vi "dll_driver.vi"(4 "position_llh":string="36.318462,138.996902,100", 6 "buffer size":i32=200000, 7 "dll state":T1(ring), 8 "error in":errorcluster, 9 "params":string, 10 "Rinex file":path=path "C:/Users/duyga/OneDrive/デスクトップ/WORKS/Nissan GPS/build dll/brdc0010.22n", 11 "dll Path":path=path "C:/Users/duyga/OneDrive/デスクトップ/WORKS/Nissan GPS/build dll/GPS_SIM_GENERATE_IQ.dll") -> (0 "error out":errorcluster, 3 "output":i16[](array[numeric]))   [LabVIEW 2020]
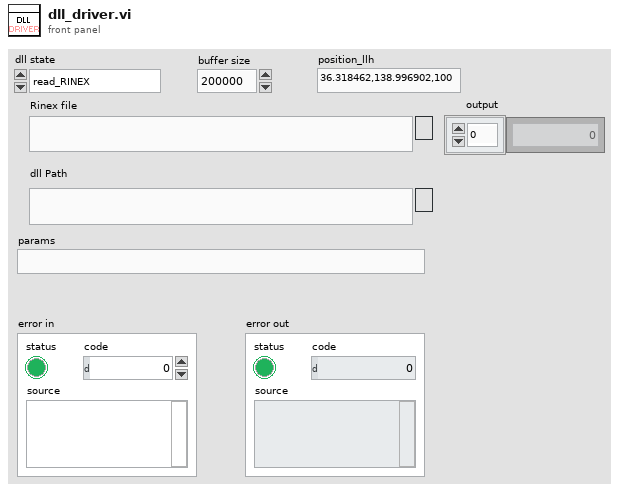
[diagram p1: front panel]
types:
  T1 = enum16{"read_RINEX", "settings", "generate_100ms", "update_position"}
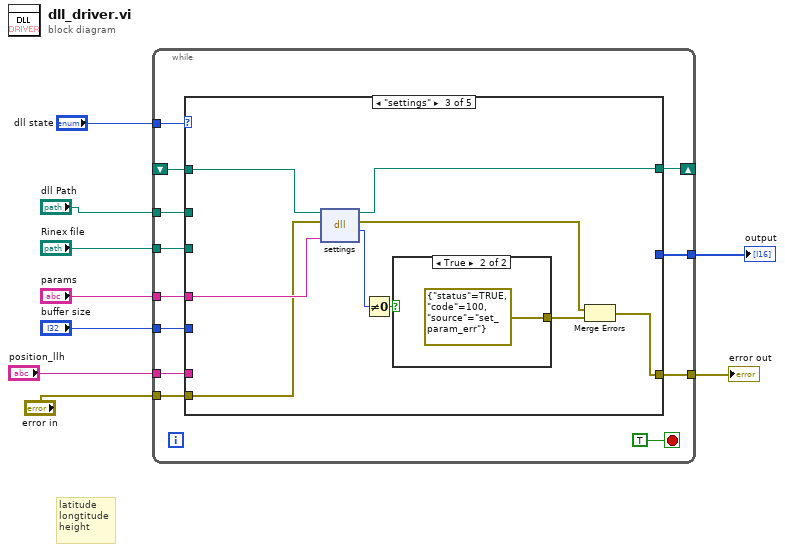
[diagram p0: block diagram]
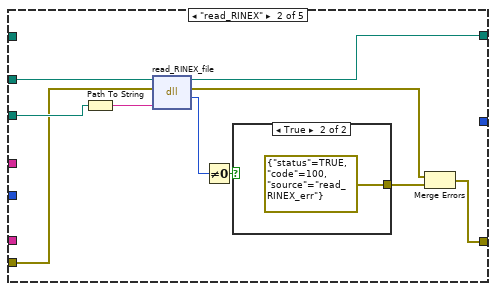
[diagram p3: hidden frame]
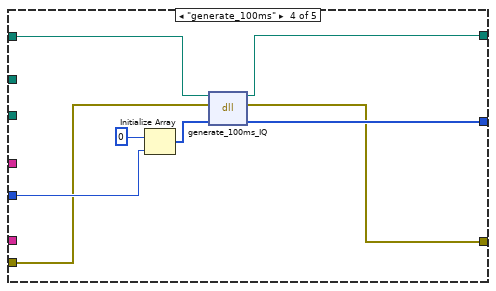
[diagram p6: hidden frame]
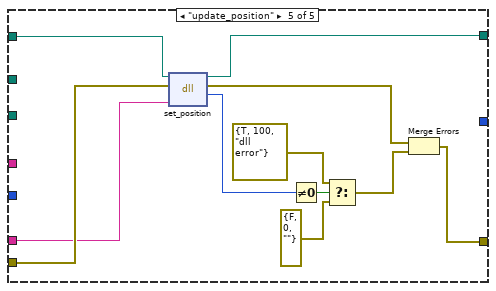
[diagram p7: hidden frame]
diagram:
  # "latitude\nlongtitude\nheight"
  n1 = while {
    tunnel: "dll state" -> [w20]
    tunnel: "dll Path" -> [w19]
    tunnel: "Rinex file" -> [w18]
    shift-right: [w17] -> _
    shift-left: _ -> [w14]
    tunnel: "error in" -> [w16]
    tunnel: [w15] -> w5
    tunnel: "params" -> [w13]
    tunnel: [w12] -> w3
    tunnel: "buffer size" -> [w11]
    tunnel: "position_llh" -> [w10]
    stop <- TRUE stop-if-true
    n2 = case shown="\"settings\"" w20 {
      tunnel: w19 -> [_ w32 _ _ _]
      tunnel: w18 -> [_ w31 _ _ _]
      tunnel: [w23 w30 w42 w47 w62] -> w17
      tunnel: w16 -> [w22 w29 w40 w45 w61]
      tunnel: [w22 w24 w35 w48 w58] -> w15
      tunnel: w14 -> [w23 _ w43 w46 w63]
      tunnel: w13 -> [_ _ w41 _ _]
      tunnel: [_ _ _ w50 _] -> w12
      tunnel: w11 -> [_ _ _ w49 _]
      tunnel: w10 -> [_ _ _ _ w53]
      frame Default {
      }
      frame "read_RINEX" {
        n3 = Path To String(path=w31) -> (string=w33:string)
        n4 = dll-call lib="PTH2mabs CUsersduygaOneDriveデスクトップWORKS\nNissan GPS\tbuild dllGPS_SIM_GENERATE_IQ_v3.DLL" fn="read_RINEX_file"(path in=w32, error in=w29, "rinex file"=w33) -> (path out=w30:path, error out=w25:errorcluster, "return"=w28:i64)  [unwired: 2 in]
        n5 = Not Equal To 0?(x=w28) -> (x != 0?=w27:bool)
        n6 = case shown="True" w27 {
          tunnel: [_ errorcluster {"status"=TRUE, "code"=100, "source"="read_RINEX_err"} ("error out")] -> w26
          frame False {
          }
          frame True {
          }
        }
        n7 = Merge Errors(w25, w26) -> (w24:errorcluster)
      }
      frame "settings" {
        n8 = dll-call lib="PTH2mabs CUsersduygaOneDriveデスクトップWORKS\nNissan GPS\tbuild dllGPS_SIM_GENERATE_IQ_v3.DLL" fn="settings"(path in=w43, error in=w40, "params"=w41) -> (path out=w42:path, error out=w36:errorcluster, "return"=w37:i64)  [unwired: 2 in]
        n9 = Not Equal To 0?(x=w37) -> (x != 0?=w39:bool)
        n10 = case shown="True" w39 {
          tunnel: [_ errorcluster {"status"=TRUE, "code"=100, "source"="set_param_err"} ("error out")] -> w38
          frame False {
          }
          frame True {
          }
        }
        n11 = Merge Errors(w36, w38) -> (w35:errorcluster)
      }
      frame "generate_100ms" {
        n12 = Initialize Array(i16 0 ("element"), w49) -> (w51:i16[])
        n13 = dll-call lib="PTH2mabs CUsersduygaOneDriveデスクトップWORKS\nNissan GPS\tbuild dllGPS_SIM_GENERATE_IQ_v3.DLL" fn="generate_100ms_IQ"(path in=w46, error in=w45, "output"=w51) -> (path out=w47:path, error out=w48:errorcluster, "output"=w50:i16[])  [unwired: 2 in]
      }
      frame "update_position" {
        n14 = dll-call lib="PTH2mabs CUsersduygaOneDriveデスクトップWORKS\nNissan GPS\tbuild dllGPS_SIM_GENERATE_IQ_v3.DLL" fn="set_position"(path in=w63, error in=w61, "str_llh"=w53) -> (path out=w62:path, error out=w59:errorcluster, "return"=w60:i64)  [unwired: 2 in]
        n15 = Not Equal To 0?(x=w60) -> (x != 0?=w57:bool)
        n16 = Select(t=errorcluster {"status"=TRUE, "code"=100, "source"="dll error"} ("error out"), s=w57, f=errorcluster {"status"=FALSE, "code"=0, "source"=""} ("error out")) -> (s? t:f=w54:errorcluster)
        n17 = Merge Errors(w59, w54) -> (w58:errorcluster)
      }
    }
  }
  "error out" <- w5
  "output" <- w3
